vi "AlliGator Source Image Profile Window.vi"() -> ()   [LabVIEW 2021, in "AlliGator Image Profile Window.lvlib"]
doc: "AlliGator Profile Window."
uses:
  AlliGator Image Profile Window.lvlib
  AlliGator Variables List.ctl
  AlliGator Source Image Profile Window Event Refnum.ctl
  AlliGator Image Profile Plot Data.ctl
  Graphs/XY Graph/XY Plot Data.ctl
  Graphs/XY Graph/XY Graph Refnum.ctl
  AlliGator Q Element.ctl
  AlliGator Q Event.ctl
  Graphs/XY Graph/XY Graph Event.ctl
  <vilib>/Utility/miscctls.llb/LVPoint32TypeDef.ctl
  Image/Box Profile Type.ctl
  Variant/Variant to Data/Variant to Boolean.vi
  Variant/Variant to Data/Variant to U32.vi
  Graphs/XY Graph/XY Graph Add-Ons.lvlib
  AlliGator Globals, Variables & Constants.lvlib
  Notebook/Notebook.lvlib
  Rich Text Box/Rich Text Box.lvlib
  AlliGator Settings.lvlib
  Image/Image.lvlib
  AlliGator Action Engine.lvlib
  Variant/Variant to Data/Variant to Data.lvlib
panel:
  out "Image Profile TipStrip":string
  out "Image Profile":cluster{"X Array":dbl[], "Y Array":dbl[]}[](graph)
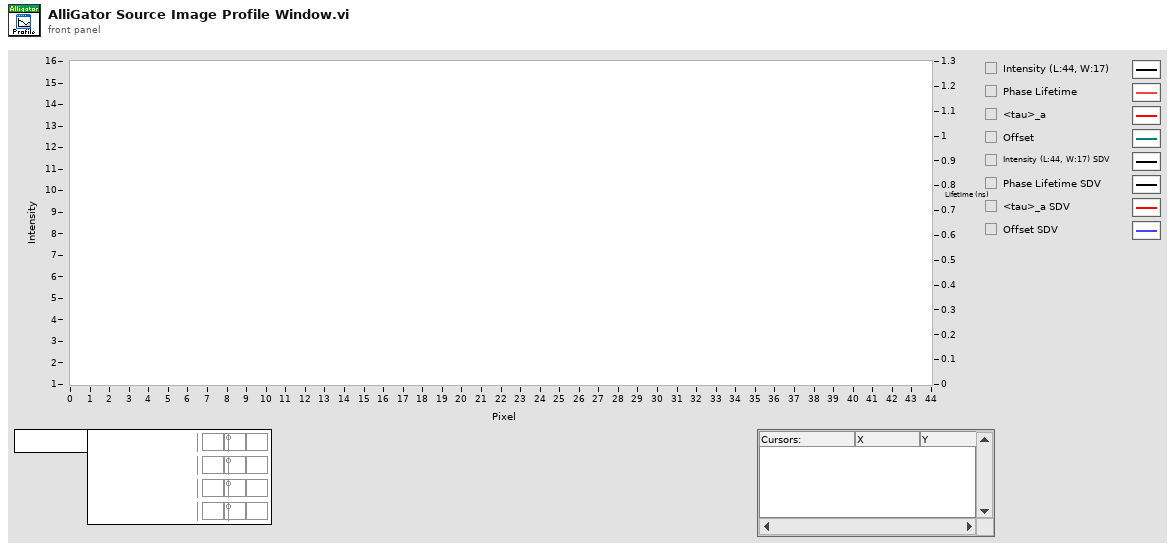
[diagram p1: front panel]
types:
  T1 = typedef "AlliGator Action Engine.lvlib/AlliGator Q Element.ctl" = cluster{"AlliGator Q Event":T2, "Data":variant}
  T2 = typedef "AlliGator Action Engine.lvlib/AlliGator Q Event.ctl" = enum16{"---- Files ----", "Files:Set Batch Export Files To Save", "Files:Set Dataset Loading & Pre-processing Options", "Files:Check #Frames in Dataset", "Files:Increment Frame Index", "Files:Open Mask Image", "Files:Open White Light Image", "Files:Open Single Dataset", "Files:New Folder of Folders Selected", "Files:Load File (all Types)_Scriptable", "Files:Move Flattened Series to Folders Series", "Files:Select Folder", "Files:Load FLI Dataset", "Files:Load Swiss SPAD 1 Dataset", "Files:Load Swiss SPAD 2 Dataset", "Files:Load .sdt FLI Dataset", "Files:Load .ptu FLI Dataset", "Files:Load .bin FLI Dataset", "Files:Load Single Gate Image Folder", "Files:Load I/m/phi Dataset (deprecated)", "Files:Load Single Image", "Files:Subtract Background File", "Files:Export FLI Dataset", "Files:Load HDF5 FLI Dataset", "Files:Set Destination File Path", "Files:Save Mask Image", "Files:Batch Conversion", "Files:New Folder Selected", "Files:Close FLI Dataset", "Files:Close FLI Dataset Series", "Files:Close White Light Image", "Files:Close Mask Image", "---- FLI Dataset ----", "FLI Dataset:Channel Arithmetic", "FLI Dataset:Export Average Lifetime Map as ASCII", "FLI Dataset:Export User-Defined Quantity Map as ASCII", "FLI Dataset:Python Function FLI Dataset Event", "FLI Dataset:ROI Analysis", "FLI Dataset:Tilted Logistic Square Gated IRF Characteristics Map", "FLI Dataset:Logistic Square Gated IRF Characteristics Map", "FLI Dataset:Square Gated IRF Characteristics Map", "FLI Dataset:Multi-ROI Single-Pixel Phasor Analysis", "FLI Dataset:Multi-ROI Single-Pixel NLSF Analysis", "FLI Dataset:All ROIs IRF Extraction", "FLI Dataset:All ROIs Decay Fit Non-Interactive (Fast + Individual IRF)", "FLI Dataset:All ROIs Phasor Analysis", "FLI Dataset:All ROIs Decay Fit", "FLI Dataset:Fluorescence Decay Statistics", "FLI Dataset:Update Decay Statistics Graph", "FLI Dataset:Get Decay from ROI", "FLI Dataset:All ROIs Average Lifetimes", "---- FLI Dataset Series ----", "FLI Dataset Series:Sum All Datasets in Series", "FLI Dataset Series:Add Dataset to Accumulated Dataset", "FLI Dataset Series:Display Accumulated Dataset", "FLI Dataset Series:Clear Dataset Series Sum", "FLI Dataset Series:Time-Series Analysis (NLSF)", "FLI Dataset Series:Time-Series Analysis (Phasor)", "---- Image ----", "Image:Update Image Profile Plots", "Image:Image Histogram Cursor Move", "Image:Image Histogram", "Image:Image Contrast", "Image:Set Image Histogram Cursor Move Flag", "Image:Clear Image Overlay", "Image:Use ROI as Search Area", "Image:Set ROI Diameter", "Image:Save Image Data as TIFF", "Image:Save Displayed Image with Overlay", "Image:Save Image Overlay Only", "Image:Save Image as Hot Pixel Mask", "Image:Change Source Image Color Palette", "Image:Copy Image to Clipboard", "Image:Source Image ROI Selection", "Image:Delete All ROIs", "Image:Delete All Unselected ROIs", "Image:Delete ROI", "Image:Merge All ROIs", "Image:Store ROI", "Image:Source Image ROI Storage", "Image:Export ROI Description to Notebook", "Image:Save ROI", "Image:Load ROI", "Image:Paste ROI Definition", "Image:Clear ROI", "Image:Identify ROIs in Mask Image", "Image:Create Complementary ROI", "Image:Create Contour ROI", "Image:Create ROI(s) from Pixels with Peak above Min_Scriptable", "Image:Create ROI(s) from Pixels with Intensity above Min_Scriptable", "Image:Compute ROI Statistics", "Image:Delete ROI(s) based on ROI Characteristics", "Image:Create ROI Grid", "Image:ROI to Individual Pixel ROIs", "Image:Python Function Source Image Event", "Image:Show Phasor Calibration Map ROI Centers", "Image:Convert ROI to Mask Image", "Image:Mouse Move", "Image:Mouse Up", "Image:Set Source Image Mouse Move Flag", "Image:Add Scale Bar Overlay", "Image:Delete Existing ROIs Option", "---- Decay ----", "Decay:Clear IRF/Reference Plot", "Decay:Clear Local IRFs", "Decay:Add Decay to Graph", "Decay:Smoothen Plot", "Decay:Smoothen Plot Tail", "Decay:Average Selected Plots", "Decay:Extract IRF", "Decay:Optimal IRF Extraction", "Decay:Threshold IRF", "Decay:Fit to Model IRF", "Decay:Fit IRF to Square Gate", "Decay:Fit IRF to Logistic Square Gate", "Decay:Fit IRF to Tilted Logistic Square Gate", "Decay:Create Bounding Cursors Set", "Decay:Export Bounding Cursors Definition to Notebook", "Decay:Denoise Plot", "Decay:Compute Cumulative Function", "Decay:Use as Reference Decay", "Decay:Show Reference Decay/IRF", "Decay:Extrapolate Decay", "Decay:Create Head & Tail Bounding Cursors", "Decay:Store Cursor-defined Head & Tail Fractions", "Decay:Rebin Plot", "Decay:1-Normalize Decay", "Decay:[0-1]-Normalize Plot", "Decay:Straighten Decay", "Decay:Shift Decay", "Decay:Fold Decay", "Decay:Fit Decay", "Decay:Global Fit of Selected Decays", "Decay:Post Global Fit Script", "Decay:Add Global Fit Parameters to Graph", "Decay:Add Decay Parameter(s) to Plot (Graph)", "Decay:Export Decay to Phasor Graph", "Decay:Plot Decay Shifts", "Decay:Compute Average Lifetime", "Decay:Plot Convolution", "Decay:Graph Tip Strip Update", "---- Decay Statistics ----", "Decay Statistics:Tip Strip Update", "---- Intensity Time Trace ----", "Intensity Time Trace:Use File Timestamp", "Intensity Time Trace:Load Intensity Corrections File", "Intensity Time Trace:Clear Intensity Corrections File", "Intensity Time Trace:Tip Strip Update", "---- Phasor Plot ----", "Phasor Plot:Build Phasor Plot", "Phasor Plot:Change Phasor Plot Color Palette", "Phasor Plot:Adjust Phasor Plot Display Range", "Phasor Plot:Highlight Image ROI in Phasor Plot", "Phasor Plot:Save Phasor Plot Image with Overlay", "Phasor Plot:Export Complex Phasor Map", "Phasor Plot:Export Phasor Ratio Map", "Phasor Plot:Export Average Lifetime Map", "Phasor Plot:Compute Phase Lifetime Histogram", "Phasor Plot:Compute Phasor Ratio Histogram", "Phasor Plot:Compute Phase Lifetime vs Intensity Scatter Plot", "Phasor Plot:Weber 2-Component Decomposition", "Phasor Plot:Update Phasor Color Map Vertices", "Phasor Plot:Clear Phasor Overlay", "Phasor Plot:Use Segment Extremities as References", "Phasor Plot:Use UC/Segment Intersections as References", "Phasor Plot:Use UC/Principal Axis Intersections as References", "Phasor Plot:Use UC/Linear Fit Intersections as References", "Phasor Plot:Update Phasor Plot Reference", "Phasor Plot:Show Local Phasor Info in Phasor Plot", "Phasor Plot:Update Phasor Plot State", "Phasor Plot:Phasor Plot ROI Storage", "Phasor Plot:Phasor Plot ROI Selection", "Phasor Plot:Python Function Phasor Plot Event", "Phasor Plot:Overlay Phasor ROI, Ratio or Map in Source Image", "Phasor Plot:Compute Decay of Selected Phasors", "Phasor Plot:Phasor at Image Pixel", "Phasor Plot:Mouse Move", "Phasor Plot:Mouse Up", "Phasor Plot:Display Range Mouse Move", "Phasor Plot:Set Mouse Move Flag", "---- Phasor Graph ----", "Phasor Graph:Calibrated Phasor Map Series", "Phasor Graph:Whole Image Phasor Scatter Plot (Todo)", "Phasor Graph:Get Phasor Value", "Phasor Graph:Create New Phasor Plot Dialog", "Phasor Graph:Update Last Phasor Value", "Phasor Graph:Update Phasor (m, phi)", "Phasor Graph:Remove Single Phasor from Plot", "Phasor Graph:Add Single Phasor to Plot", "Phasor Graph:Remove Phasor Plot", "Phasor Graph:Remove Selected Phasor Plots", "Phasor Graph:Clear Phasor Data", "Phasor Graph:Clear Phasor Graph", "Phasor Graph:Cursor Move", "Phasor Graph:Draw Cursor Connecting Line", "Phasor Graph:Clear Cursor Connecting Line", "Phasor Graph:Find UC Intersection", "Phasor Graph:Use UC/Cursor-Defined Line Intersections", "Phasor Graph:Use Selected Plots Fitted Line/UC Intersections", "Phasor Graph:Use Selected Plots Principal Axis/UC Intersections", "Phasor Graph:Show Single Phasor", "Phasor Graph:Save Single Phasor Plot", "Phasor Graph:Save All Phasor Plots", "Phasor Graph:Load Phasor Plot(s)", "Phasor Graph:Phasor Multiplication", "Phasor Graph:Compute Average Phasor", "Phasor Graph:Compute Multiple Average Phasors (Selected Plots)", "Phasor Graph:Export Single Phasor Plot Phase Lifetimes", "Phasor Graph:Phase Lifetime Trajectory", "Phasor Graph:Phase Lifetime vs Intensity Scatter Plot (deprecated)", "Phasor Graph:Parameter 2 vs Parameter 1 Scatter Plot", "Phasor Graph:Use Cursor n Location", "Phasor Graph:Set Reference n to Current Phase Lifetime Value", "Phasor Graph:Set Reference n to Lifetime Value", "Phasor Graph:Set Cursor n Location", "Phasor Graph:Save Phasor Graph Image", "Phasor Graph:Update SEPL Plot", "Phasor Graph:Export Single Phasor Plot Data", "Phasor Graph:Export Selected Phasor Plots Data", "Phasor Graph:Python Function Phasor Graph Event", "Phasor Graph:Tip Strip Update", "---- Calibration ----", "Calibration:Set Calibration Type", "Calibration:Load/Save Phasor Calibration", "Calibration:Load/Save Phasor Calibration Series", "Calibration:Load/Save Phasor Calibration Map", "Calibration:Use as Calibration", "Calibration:Compute Optimal Calibration from Phasor References", "Calibration:Clear Phasor Calibration", "Calibration:Single Phasor Calibration Information", "Calibration:Use as Calibration Series", "Calibration:Use as Calibration Map", "Calibration:Clear Calibration Series", "Calibration:Phasor Calibration Series Information", "Calibration:Clear Calibration Map", "Calibration:Phasor Calibration Map Information", "Calibration:Apply Phasor Calibration", "Calibration:Update Single Plot Calibration", "Calibration:Update Multiple Plots Calibration", "Calibration:Clear Single Plot Calibration", "Calibration:Clear All Plots Calibrations", "Calibration:Clear Plot(s) Calibration(s)?", "Calibration:Phasor Calibration Maps (# Gates Series)", "---- Phasor Ratio ----", "Phasor Ratio:Clear Reference n", "Phasor Ratio:Toggle Selected Plot(s)  Lock to Reference 1", "Phasor Ratio:Use as Reference n", "Phasor Ratio:Send Reference n to Notebook", "Phasor Ratio:Toggle Selected Plot(s)  Lock to Reference 2", "Phasor Ratio:Compute Phasor Ratio at Mouse Location", "Phasor Ratio:Compute Phasor Plot's Average Phasor Ratio", "Phasor Ratio:Compute Time-Series Phasor Ratios", "Phasor Ratio:Fit Line to Phasor Ratio Plot", "Phasor Ratio:Save References", "Phasor Ratio:Load References", "Phasor Ratio:Update Phasor Reference 1", "Phasor Ratio:Update Phasor Reference 2", "Phasor Ratio:Move Cursor n to Reference n", "Phasor Ratio:Use as Phasor Reference 1 Lifetime", "Phasor Ratio:Use as Phasor Reference 2 Lifetime", "Phasor Ratio:Export Phasor Ratio Map as ASCII", "Phasor Ratio:Tip Strip Update", "---- Lifetime & Other Parameters Graph ----", "Lifetime:Tip Strip Update", "---- Decay Fit Parameter Map ----", "Decay Fit Parameter Map:Export ROI NLSF Data as ASCII", "Decay Fit Parameter Map:Set Decay Fit  Parameter Map Selection", "Decay Fit Parameter Map:Build Decay Fit Parameter Map", "Decay Fit Parameter Map:Change Decay Fit Parameter Map Color Palette", "Decay Fit Parameter Map:Export Decay Fit Parameter Map Data as ASCII", "Decay Fit Parameter Map:Export All Decay Fit Parameter Maps Data as ASCII", "Decay Fit Parameter Map:Send Map Data to Lifetime Graph", "Decay Fit Parameter Map:Save Decay Fit Parameter Map Image", "Decay Fit Parameter Map:Save-Load IRFs & Fit Data", "Decay Fit Parameter Map:Update Local Decay Plots", "Decay Fit Parameter Map:Python Function Decay Fit Parameters Map Event", "Decay Fit Parameter Map:Overlay Decay Fit Parameter Map in Source Image", "Decay Fit Parameter Map:Plot Map Data vs Intensity", "Decay Fit Parameter Map:Mouse Up", "Decay Fit Parameter Map:Display Range Mouse Move", "---- Generic Graph ----", "Generic Graph:Generic XY Graph Event", "Generic Graph:Python Function XY Graph Event", "Generic Graph:New Plot", "Generic Graph:Save Plot", "Generic Graph:XY Plot Histogram", "Generic Graph:Set XY Graph Plot Name", "Generic Graph:Set Last Cursor Style", "Generic Graph:Tip Strip Update", "---- GUI ----", "GUI:Start Script", "GUI:Type of Displayed Image Changed", "GUI:Gate Image Slide Changed", "GUI:Show Busy Icon", "GUI:Show Busy Icon & Abort Button", "GUI:Hide Busy Icon", "GUI:Hide Busy Icon & Abort Button", "GUI:Abort", "GUI:End Script", "GUI:Start Timing", "GUI:End Timing", "GUI:Set State Indicator", "GUI:Send Parameters JSON Strings to Clipboard", "GUI:Set Gate Step", "GUI:Idle", "GUI:Initialization", "GUI:Quit", "GUI:Increment Dataset Index", "GUI:Set Dataset Index to -1", "GUI:Time Series Slider Moved", "GUI:Time Series Slider Changed", "GUI:Toggle Playback or Loop", "GUI:Playback Script", "GUI:Set Phasor Frequency", "GUI:Open Window", "GUI:Start Test Script", "GUI:End Test Script", "DEBUG"}
  T3 = typedef "AlliGator Globals, Variables & Constants.lvlib/AlliGator Variables List.ctl" = enum16{"---- GUI ----", "Initialization Status", "State Indicators Refnum", "Original AlliGator Menu Items", "Current Action Loop State", "Script in progress", "Playback", "Loop Playback", "Search ROI Used", "Search ROI", "Decay Graph Max Legend Size", "Intensity Graph Max Legend Size", "Decay Statistics Graph Max Legend Size", "Phasor Graph Max Legend Size", "Phasor Ratio Graph Max Legend Size", "Lifetime Graph Max Legend Size", "---- Files ----", "Export Dataset Frames as Individual Files", "Show Batch Export Help Balloons", "Frames in Dataset", "ptu File Frame Start Indices", "Current Frame in Dataset", "Current Frame Timestamp", "------ Python Plugins ------", "Python Plugins Information", "Python Session", "Valid Python Session?", "---- Source Image ----", "Dataset Loaded", "Dataset Metadata", "Dataset Channel", "Dataset Data Description", "Background Dataset Metadata", "Background Dataset Channel", "Background Dataset Data Description", "Background File Subtraction", "Background File Path", "Background File Pile-up Correction", "Background File Pixel Well Capacity", "Background File Scaling Factor", "Source Image ROIs", "Current Source Image ROI", "Source Image ROI Event Refnum", "X_Source Image Display Range", "X_Source Image Palette Information", "Source Image Palette List", "Source Image Scale", "Current Dataset Load Settings", "Source Image:ROI Overlay Color", "---- Image Profile Window ----", "Image Profile:Overlay ROI in Source Image", "Image Profile Window Event Refnum", "Image Profile:IntensityType", "Image Profile:Intensity Average Type", "Image Profile:Intensity-weighted SDV", "Image Profile:Box Profile Type", "Image Profile Window Open", "Image Profile:Plotted Fit Parameter", "X_Type of Displayed Image", "X_Time Gate Slider", "Dataset Path", "Source Image Overlay to Erase", "Is Displayed Image Accumulated", "White Light Image Modified", "Mask Image Modified", "Macrotime Gate Separation", "------ Phasor Graph -------", "Phasor Graph:Show Line", "---- Phasor Plot ---", "Phasor Plot Parameters Changed", "FLI Dataset Modified since last Phasor Plot Calculation", "Phasor Harmonics Data", "Selected Phasor Harmonics", "Phasor Harmonic Manager Event Refnum", "Phasor Plot ROIs", "Current Phasor Plot ROI", "Phasor Plot ROI Event Refnum", "Phasor Plot Image Reference Points", "Phasor Plot Computed", "Phasor Plot Palette Information", "Phasor Plot Palette List", "Phasor Ratio Palette Information", "Phasor Ratio Palette List", "Phasor Image Scale", "Phasor Plot Image Overlay to Erase", "Phasor Plot Image Elements to Update", "Current Phasor Plot Calculation Parameters", "Current Phasor Calibration Options", "Reset Cumulated Phasor Plot", "Phasor Ratio Reference 1", "Phasor Ratio Lifetime Reference 1", "Phasor Ratio Reference 1 Frequency", "Phasor Ratio Reference 2", "Phasor Ratio Lifetime Reference 2", "Phasor Ratio Reference 2 Frequency", "---- Decay Analysis ----", "Number of Selected Decays to Fit", "LS Fit Results", "LAR Fit Results", "BS Fit Results", "Last Decay Max - Min", "Best Fit Parameters", "Best Fit Parameter Names", "Actual Size X", "Actual Size Y", "Binning X", "Binning Y", "Actual # Gates", "Dataset Number", "Gates to...", "Gates Skipped", "Gates to keep", "Gate Step", "Gate Separation", "Reversed Gates", "Pile-up Correction", "Pixel Well Capacity", "Background Subtracted", "Background Subtraction Method", "Background Definition Range", "Background File (deprecated)", "Number of Dataset Accumulated", "Array of Accumulated Dataset Paths", "Do Averaged Datasets", "Destination File Path", "Process Plot Target", "Use 1/D as Phasor Frequency", "---- Decay Fit Parameter Map -----", "Decay Fit Parameter Map Palette Information", "Decay Fit Parameter Map Palette List", "Local Decay Graph Window Event Refnum", "------- Local Decay Window ---------", "Use normalized IRF for convolution", "----- Miscellaneous ----", "Skippable Dialog Windows Status"}
  T4 = cluster{"Image Profile TipStrip Event":refnum<event-registration>, "Source Image Profile Window Event":refnum<event-registration>}
  T5 = typedef "AlliGator Image Profile Window.lvlib/AlliGator Source Image Profile Window Event Refnum.ctl" = refnum<user-event>
  T6 = enum32{"Invalid", "Standard", "Closed", "Hidden", "Minimized", "Maximized"}
  T7 = typedef "XY Graph Add-Ons.lvlib/XY Graph Refnum.ctl" = refnum<vi>
  T8 = typedef "XY Graph Add-Ons.lvlib/XY Graph Event.ctl" = cluster{"Item Tag":string, "XY Graph Refnum":refnum<vi>, "Coords":T9, "Item Path":string}
  T9 = typedef "LVPoint32TypeDef.ctl" = cluster{"Horizontal":i32, "Vertical":i32}
  T10 = typedef "Image.lvlib/Box Profile Type.ctl" = enum16{"Full Width", "Half Width"}
  T11 = typedef "Rich Text Box.lvlib/Text Formatting.ctl" = cluster{"Font":string, "Text Color":T12, "Text Background Color":T12, "Text Style":enum16{"Regular", "Bold", "Italic", "Underline", "Strikeout"}, "Font Size (Points)":dbl, "Text Alignment":i32}
  T12 = typedef "Rich Text Box.lvlib/Text Colors.ctl" = enum16{"Unchanged", "Black", "Blue", "Brown", "Gray", "Green", "Orange", "Pink", "Red", "White"}
  T13 = typedef "AlliGator Image Profile Window.lvlib/AlliGator Image Profile Plot Data.ctl" = cluster{"Plot Name":string, "Plot":T14}
  T14 = typedef "XY Graph Add-Ons.lvlib/XY Plot Data.ctl" = cluster{"X Array":dbl[], "Y Array":dbl[]}
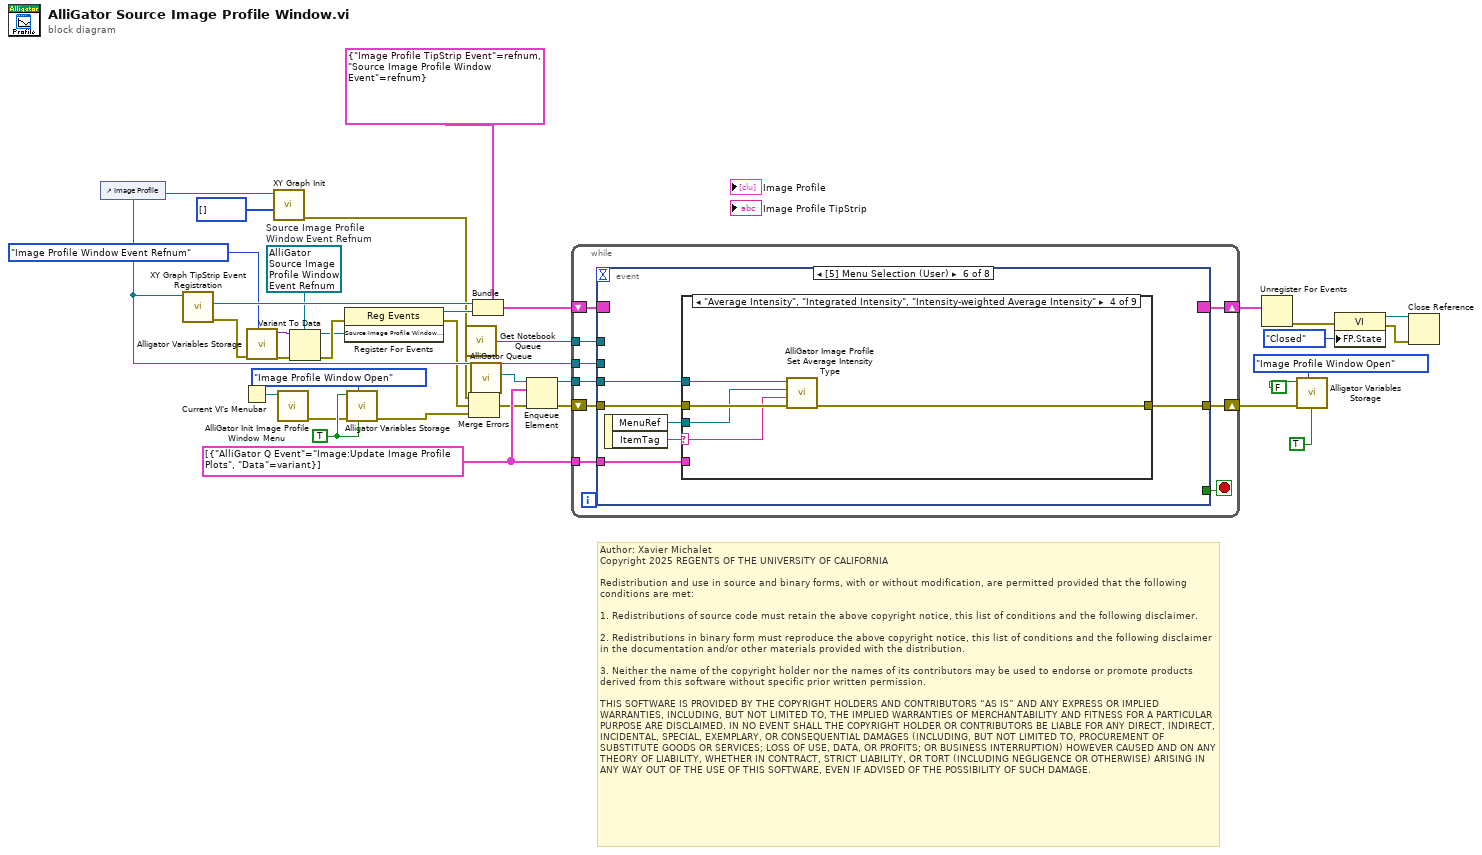
[diagram p0: block diagram]
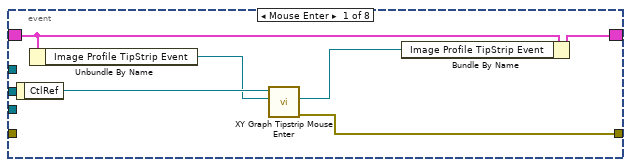
[diagram p2: hidden frame]
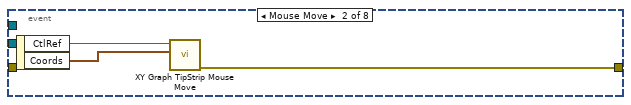
[diagram p3: hidden frame]
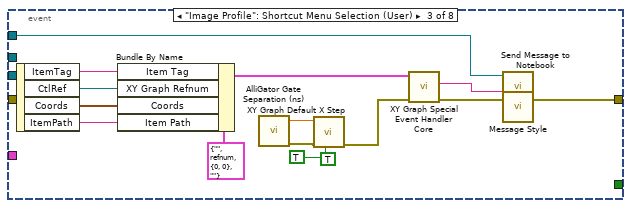
[diagram p4: hidden frame]
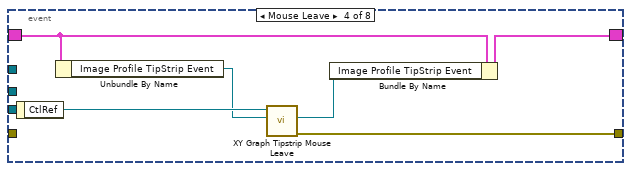
[diagram p5: hidden frame]
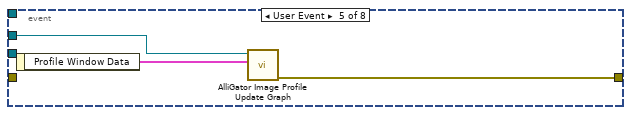
[diagram p6: hidden frame]
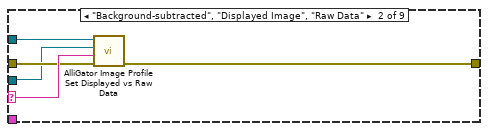
[diagram p8: hidden frame]
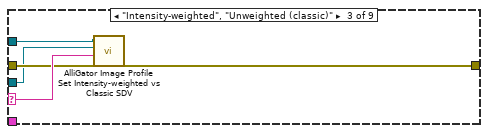
[diagram p9: hidden frame]
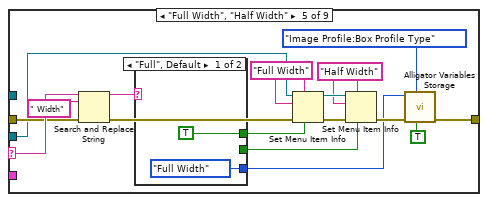
[diagram p10: hidden frame]
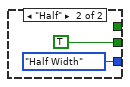
[diagram p11: hidden frame]
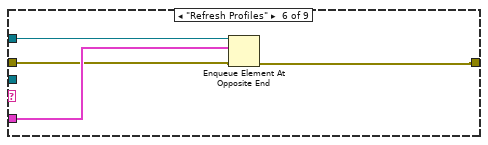
[diagram p12: hidden frame]
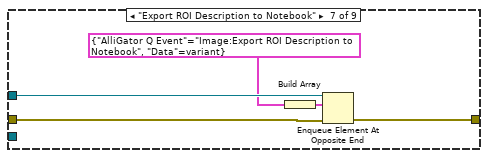
[diagram p13: hidden frame]
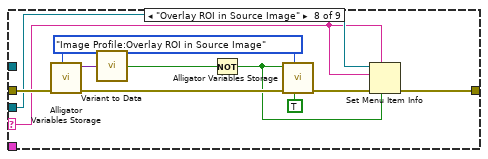
[diagram p14: hidden frame]
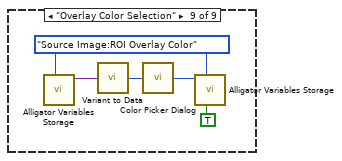
[diagram p15: hidden frame]
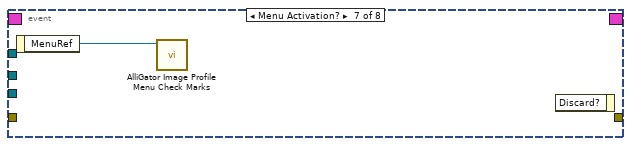
[diagram p16: hidden frame]
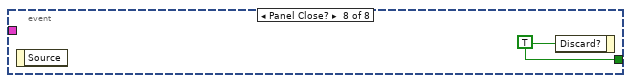
[diagram p17: hidden frame]
diagram:
  w3 = T1[] [{"AlliGator Q Event"=enum."Image:Update Image Profile Plots", "Data"=variant}] ("element")
  w11 = TRUE (".not. x?")
  w24 = T5 refnum  # Source Image Profile Window Event Refnum
  # "Author: Xavier Michalet\nCopyright 2025 REGENTS OF THE UNIVERSITY OF CALIFORNIA\n\nRedistribution and use in source and binary forms, with or without modification, are permitted provided that the following conditions are met:\n\n1. Redistributions of source code must retain the above copyright notice, this list of conditions and the following disclaimer.\n\n2. Redistributions in binary form must reproduce the above copyright notice, this list of conditions and the following disclaimer in the documentation and/or other materials provided with the distribution.\n\n3. Neither the name of the copyright holder nor the names of its contributors may be used to endorse or promote products derived from this software without specific prior written permission.\n\nTHIS SOFTWARE IS PROVIDED BY THE COPYRIGHT HOLDERS AND CONTRIBUTORS “AS IS” AND ANY EXPRESS OR IMPLIED WARRANTIES, INCLUDING, BUT NOT LIMITED TO, THE IMPLIED WARRANTIES OF MERCHANTABILITY AND FITNESS FOR A PARTICULAR PURPOSE ARE DISCLAIMED. IN NO EVENT SHALL THE COPYRIGHT HOLDER OR CONTRIBUTORS BE LIABLE FOR ANY DIRECT, INDIRECT, INCIDENTAL, SPECIAL, EXEMPLARY, OR CONSEQUENTIAL DAMAGES (INCLUDING, BUT NOT LIMITED TO, PROCUREMENT OF SUBSTITUTE GOODS OR SERVICES; LOSS OF USE, DATA, OR PROFITS; OR BUSINESS INTERRUPTION) HOWEVER CAUSED AND ON ANY THEORY OF LIABILITY, WHETHER IN CONTRACT, STRICT LIABILITY, OR TORT (INCLUDING NEGLIGENCE OR OTHERWISE) ARISING IN ANY WAY OUT OF THE USE OF THIS SOFTWARE, EVEN IF ADVISED OF THE POSSIBILITY OF SUCH DAMAGE."
  n1 = control-ref of="Image Profile"() -> (w28:refnum<vi>)
  n2 = call "XY Graph TipStrip Event Registration.vi"("XY Graph Refnum"=w28) -> ("error out"=w16:errorcluster, "Event Registration Refnum"=w34:refnum<event-registration>, "XY Graph Refnum"=w29:T7)  [unwired: 8 in]
  n3 = Current VI's Menubar() -> (w9:refnum<k9>)
  n4 = call "Alligator Variables Storage.vi"("AlliGator Variable"=AlliGator_Variables_List."Image Profile Window Event Refnum" ("Alligator Variable"), "Error In"=w16) -> ("Error Out"=w25:errorcluster, "Data out"=w26:variant)  [unwired: 7 in, 1 out]
  n5 = call "XY Graph Init.vi"("Plots to Skip (none)"=i32[] [], "XYGraph in"=w29) -> ("Error Out"=w15:errorcluster)  [unwired: 9 in]
  n6 = call "AlliGator Init Image Profile Window Menu.vi"("Menu in"=w9) -> ("error out"=w8:errorcluster)  [unwired: 10 in]
  n7 = Variant To Data(error in=w25, type=w24, Variant=w26) -> (data=w22:T5, error out=w23:errorcluster)
  n8 = register-events(error in=w23, w22) -> (reference out=w21:refnum<event-registration>, error out=w17:errorcluster)  [unwired: 1 in]
  n9 = call "Alligator Variables Storage.vi"("Get(F)/Set"=w11, "AlliGator Variable"=AlliGator_Variables_List."Image Profile Window Open" ("Alligator Variable"), "Error In"=w8, "Data in"=w11) -> ("Error Out"=w14:errorcluster)  [unwired: 5 in, 2 out]
  n10 = call "Get Notebook Queue.vi"() -> ("Notebook Queue"=w18:refnum<queue>)  [unwired: 9 in]
  n11 = Merge Errors(w15, w17, w14) -> (w1:errorcluster)
  n12 = call "AlliGator Queue.vi"() -> ("AlliGator Q"=w5:refnum<queue>)  [unwired: 8 in, 1 out]
  n13 = Bundle(cluster=T4 {"Image Profile TipStrip Event"=refnum, "Source Image Profile Window Event"=refnum}, "Image Profile TipStrip Event"=w34, "Source Image Profile Window Event"=w21) -> (w19:T4)
  n14 = Enqueue Element(queue=w5, element=w3, error in (no error)=w1) -> (queue out=w4:refnum<queue>, error out=w2:errorcluster)  [unwired: 1 in, 1 out]
  n15 = while {
    shift-right: [w44] -> w35
    shift-left: w19 -> [w45]
    tunnel: w28 -> [w43]
    tunnel: w18 -> [w42]
    shift-right: [w41] -> w13
    shift-left: w2 -> [w39]
    tunnel: w4 -> [w38]
    tunnel: w3 -> [w37]
    stop <- w40 stop-if-true
    n16 = event shown="[5] Menu Selection (User)" {
      selector: w45 -> [w49 _ _ w72 _ _ _ _]
      dyn-events: [w51 _ _ w71 _ _ _ _] -> w44
      timeout: _ -> [_ _ _ _ _ _ _ _]
      tunnel: [_ _ _ _ _ _ _ w148] -> w40
      tunnel: w43 -> [_ _ _ _ w78 _ _ _]
      tunnel: w42 -> [_ _ w67 _ _ _ _ _]
      tunnel: [w46 w52 w65 w70 w77 w82 _ _] -> w41
      tunnel: w39 -> [_ _ _ _ _ w81 _ _]
      tunnel: w38 -> [_ _ _ _ _ w80 _ _]
      tunnel: w37 -> [_ _ _ _ _ w79 _ _]
      event Mouse Enter {
        n17 = event-data() -> ("CtlRef"=w50:refnum<vi>)  [unwired: 1 in]
        n18 = Unbundle By Name(w49) -> ("Image Profile TipStrip Event"=w48:refnum<event-registration>)
        n19 = call "XY Graph Tipstrip Mouse Enter.vi"("Event Registration Refnum"=w48, "XY Graph Refnum"=w50) -> ("Error Out"=w46:errorcluster, "Event Registration Refnum"=w47:refnum<event-registration>)  [unwired: 8 in]
        n20 = Bundle By Name(cluster=w49, "Image Profile TipStrip Event"=w47) -> (w51:T4)
      }
      event Mouse Move {
        n21 = event-data() -> ("CtlRef"=w54:refnum<vi>, "Coords"=w53:T9)  [unwired: 1 in]
        n22 = call "XY Graph TipStrip Mouse Move.vi"("Coords"=w53, "XY Graph Refnum"=w54) -> ("Error Out"=w52:errorcluster)  [unwired: 7 in, 2 out]
      }
      event "Image Profile": Shortcut Menu Selection (User) {
        (unwired) TRUE ("Get (F)/Set")
        n23 = event-data() -> ("ItemTag"=w64:string, "CtlRef"=w63:refnum<vi>, "Coords"=w62:T9, "ItemPath"=w61:string)  [unwired: 1 in]
        n24 = Bundle By Name(cluster=T8 {"Item Tag"="", "XY Graph Refnum"=refnum, "Coords"={"Horizontal"=0, "Vertical"=0}, "Item Path"=""} ("XY Graph Event"), "Item Tag"=w64, "XY Graph Refnum"=w63, "Coords"=w62, "Item Path"=w61) -> (w59:T8)
        n25 = call "AlliGator Gate Separation (ns).vi"() -> ("error out"=w58:errorcluster, "Gate Separation (ns)"=w56:dbl)  [unwired: 10 in]
        n26 = call "XY Graph Default X Step.vi"("Get (F)/Set"=TRUE, "Error In"=w58, "Default X Step"=w56) -> ("Error Out"=w57:errorcluster)  [unwired: 7 in, 1 out]
        n27 = call "XY Graph Special Event Handler Core.vi"("error in (no error)"=w57, "XY Graph Event"=w59) -> ("error out"=w69:errorcluster, "Message"=w68:string)  [unwired: 5 in, 3 out]
        n28 = call "Message Style.vi"() -> ("Message Formatting"=w66:T11)
        n29 = call "Send Message to Notebook.vi"("Text Formatting"=w66, "Error In"=w69, "Message"=w68, "Notebook Queue"=w67) -> ("Error Out"=w65:errorcluster)  [unwired: 4 in, 1 out]
      }
      event Mouse Leave {
        n30 = event-data() -> ("CtlRef"=w75:refnum<vi>)  [unwired: 1 in]
        n31 = Unbundle By Name(w72) -> ("Image Profile TipStrip Event"=w74:refnum<event-registration>)
        n32 = call "XY Graph Tipstrip Mouse Leave.vi"("Event Registration Refnum"=w74, "XY Graph Refnum"=w75) -> ("Error Out"=w70:errorcluster, "Event Registration Refnum"=w73:refnum<event-registration>)  [unwired: 8 in]
        n33 = Bundle By Name(cluster=w72, "Image Profile TipStrip Event"=w73) -> (w71:T4)
      }
      event User Event {
        n34 = event-data() -> ("Profile Window Data"=w76:T13[])  [unwired: 1 in]
        n35 = call "AlliGator Image Profile Update Graph.vi"("Profile Window Data"=w76, "XY Graph Refnum"=w78) -> ("Error Out"=w77:errorcluster)  [unwired: 9 in]
      }
      event Menu Selection (User) {
        n36 = event-data() -> ("MenuRef"=w84:refnum<k9>, "ItemTag"=w83:string)  [unwired: 1 in]
        n37 = case shown="\"Average Intensity\", \"Integrated Intensity\", \"Intensity-weighted Average Intensity\"" w83 {
          selector: w83 -> [_ w90 w95 w97 w117 _ _ w134 _]
          tunnel: w84 -> [_ w87 w92 w96 w101 _ _ w135 _]
          tunnel: [w85 w89 w94 w98 w105 w123 w128 w132 _] -> w82
          tunnel: w81 -> [w85 w88 w93 w99 w108 w122 w129 w141 _]
          tunnel: w80 -> [_ w86 w91 w100 _ w125 w130 _ _]
          tunnel: w79 -> [_ _ _ _ _ w124 _ _ _]
          frame "", Default {
          }
          frame "Background-subtracted", "Displayed Image", "Raw Data" {
            n38 = call "AlliGator Image Profile Set Displayed vs Raw Data.vi"("Error In"=w88, "ItemTag"=w90, "Menu in"=w87, "AlliGator Queue"=w86) -> ("Error Out"=w89:errorcluster)  [unwired: 7 in]
          }
          frame "Intensity-weighted", "Unweighted (classic)" {
            n39 = call "AlliGator Image Profile Set Intensity-weighted vs Classic SDV.vi"("Error In"=w93, "ItemTag"=w95, "Menu in"=w92, "AlliGator Queue"=w91) -> ("Error Out"=w94:errorcluster)  [unwired: 7 in]
          }
          frame "Average Intensity", "Integrated Intensity", "Intensity-weighted Average Intensity" {
            n40 = call "AlliGator Image Profile Set Average Intensity Type.vi"("Error In"=w99, "ItemTag"=w97, "Menu in"=w96, "AlliGator Queue"=w100) -> ("Error Out"=w98:errorcluster)  [unwired: 7 in]
          }
          frame "Full Width", "Half Width" {
            w110 = "Half Width" ("item tag")
            w111 = "Full Width" ("item tag")
            n41 = Search and Replace String(input string=w117, search string=" Width", error in=w108) -> (result string=w115:string, error out=w107:errorcluster)  [unwired: 5 in, 2 out]
            n42 = case shown="\"Full\", Default" w115 {
              tunnel: [TRUE ("checked") _] -> w114
              tunnel: [_ TRUE ("checked")] -> w112
              tunnel: [Box_Profile_Type."Full Width" Box_Profile_Type."Half Width"] -> w104
              frame "Full", Default {
              }
              frame "Half" {
              }
            }
            n43 = Set Menu Item Info(6:w114, 7:w111, 8:w107, 10:w111, 11:w101) -> (0:w109:errorcluster, 3:w113:refnum<k9>)  [unwired: 2 in]
            n44 = Set Menu Item Info(6:w112, 7:w110, 8:w109, 10:w110, 11:w113) -> (0:w106:errorcluster)  [unwired: 2 in, 1 out]
            n45 = call "Alligator Variables Storage.vi"("Get(F)/Set"=TRUE, "AlliGator Variable"=AlliGator_Variables_List."Image Profile:Box Profile Type" ("Alligator Variable"), "Error In"=w106, "Data in"=w104) -> ("Error Out"=w105:errorcluster)  [unwired: 5 in, 2 out]
          }
          frame "Refresh Profiles" {
            n46 = Enqueue Element At Opposite End(queue=w125, element=w124, error in (no error)=w122) -> (error out=w123:errorcluster)  [unwired: 1 in, 2 out]
          }
          frame "Export ROI Description to Notebook" {
            n47 = Build Array(T1 {"AlliGator Q Event"=enum."Image:Export ROI Description to Notebook", "Data"=variant} ("Time-Gated Phasor Q Element")) -> (w127:T1[])
            n48 = Enqueue Element At Opposite End(queue=w130, element=w127, error in (no error)=w129) -> (error out=w128:errorcluster)  [unwired: 1 in, 2 out]
          }
          frame "Overlay ROI in Source Image" {
            w140 = AlliGator_Variables_List."Image Profile:Overlay ROI in Source Image" ("Alligator Variable")
            n49 = call "Alligator Variables Storage.vi"("AlliGator Variable"=w140, "Error In"=w141) -> ("Error Out"=w139:errorcluster, "Data out"=w138:variant)  [unwired: 7 in, 1 out]
            n50 = call-poly "Variant to Data.vi"("Variant"=w138) -> ("Value"=w137:bool)  [unwired: 8 in]
            n51 = Not(x=w137) -> (.not. x?=w133:bool)
            n52 = call "Alligator Variables Storage.vi"("Get(F)/Set"=TRUE, "AlliGator Variable"=w140, "Error In"=w139, "Data in"=w133) -> ("Error Out"=w136:errorcluster)  [unwired: 5 in, 2 out]
            n53 = Set Menu Item Info(6:w133, 7:w134, 8:w136, 10:w134, 11:w135) -> (0:w132:errorcluster)  [unwired: 2 in, 1 out]
          }
          frame "Overlay Color Selection" {
            w145 = AlliGator_Variables_List."Source Image:ROI Overlay Color" ("Alligator Variable")
            n54 = call "Alligator Variables Storage.vi"("AlliGator Variable"=w145) -> ("Data out"=w144:variant)  [unwired: 8 in, 2 out]
            n55 = call-poly "Variant to Data.vi"("Variant"=w144) -> ("Value"=w143:u32)  [unwired: 8 in]
            n56 = call "Color Picker Dialog.vi"("Color in (Unchanged)"=w143) -> ("Selected Color"=w142:u32)
            n57 = call "Alligator Variables Storage.vi"("Get(F)/Set"=TRUE, "AlliGator Variable"=w145, "Data in"=w142) -> ()  [unwired: 6 in, 3 out]
          }
        }
      }
      event Menu Activation? {
        n58 = event-data() -> ("MenuRef"=w147:refnum<k9>)  [unwired: 1 in]
        n59 = call "AlliGator Image Profile Menu Check Marks.vi"("Menu in"=w147) -> ()  [unwired: 10 in, 1 out]
        n60 = event-data() -> ()  [unwired: 2 in, 1 out]
      }
      event Panel Close? {
        w148 = TRUE ("Discard?")
        n61 = event-data() -> ()  [unwired: 1 in, 1 out]
        n62 = event-data("Discard?"=w148) -> ()  [unwired: 1 in, 1 out]
      }
    }
  }
  n63 = Unregister For Events(event registration refnum=w35) -> (error out=w33:errorcluster)  [unwired: 1 in]
  n64 = call "Alligator Variables Storage.vi"("Get(F)/Set"=TRUE (".not. x?"), "AlliGator Variable"=AlliGator_Variables_List."Image Profile Window Open" ("Alligator Variable"), "Error In"=w13, "Data in"=FALSE (".not. x?")) -> ()  [unwired: 5 in, 3 out]
  n65 = property class="VI"(error in=w33, "FP.State"=T6."Closed" ("Front Panel Window:State")) -> (reference out=w31:refnum<vi>, error out=w30:errorcluster)  [unwired: 1 in]
  n66 = Close Reference(reference=w31, error in (no error)=w30) -> ()  [unwired: 1 out]
